vi "G4BaseTemplate_Singleton_6x8x6_GetProperty.vi"(5 "Error In":errorcluster) -> (16 "Property":dbl, 19 "Error Out":errorcluster)   [LabVIEW 2020]
uses:
  G4BaseTemplate_Singleton_6x8x6.lvclass
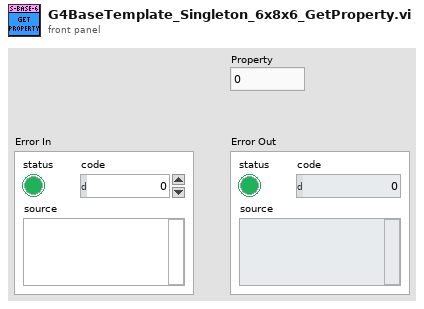
[diagram p1: front panel]
types:
  T1 = typedef "G4BaseTemplate_Singleton_6x8x6.lvclass/ObjectAttributes.ctl" = cluster{"Attribute1":dbl}
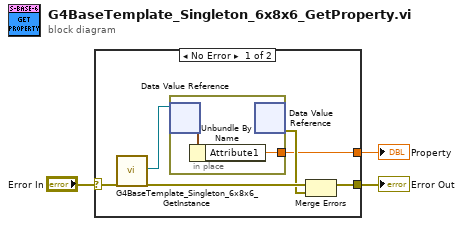
[diagram p0: block diagram]
diagram:
  n1 = case shown="No Error" "Error In" {
    selector: "Error In" -> [w9 w12]
    tunnel: [w7 w12] -> w2
    tunnel: [w5 _] -> w1
    frame No Error {
      n2 = call "G4BaseTemplate_Singleton_6x8x6_GetInstance.vi"("Error In"=w9) -> ("DVRRefOut"=w4:refnum<data-value>, "Error Out"=w8:errorcluster)  [unwired: 14 in, 3 out]
      n3 = in-place {
        in-place-border: [w11] -> w5
        n4 = in-place-dvr #1(w4) -> (w10:T1)  [unwired: 1 out]
        n5 = Unbundle By Name(w10) -> ("Attribute1"=w11:dbl)
        n6 = in-place-dvr #1() -> (w6:errorcluster)  [unwired: 1 in, 1 out]
      }
      n7 = Merge Errors(w8, w6) -> (w7:errorcluster)
    }
    frame Error {
    }
  }
  "Error Out" <- w2
  "Property" <- w1
